vi "Msg Receive.vi"(11 "Self Actor in":refnum<class "Self Actor.lvclass">) -> (0 "error out":errorcluster, 2 "Destroy Self?":bool, 3 "Msg Receive out":refnum<class "Msg Receive.lvclass">)   [LabVIEW 2021, in "AAM.lvlib" / "Self Actor.lvclass"]
uses:
  Self Actor.lvclass
  C:/PPLs/LabVIEW-Composed-Actor-Model-LVCAM/LabVIEW-Composed-Actor-Model-LVCAM/AAM/AAM/Actor/Actor.lvclass
  Msg Receive/Msg Receive.lvclass
  Self Actor.lvclass/Self Actor.ctl
  Actor/Actor.lvclass
  C:/PPLs/LabVIEW-Composed-Actor-Model-LVCAM/LabVIEW-Composed-Actor-Model-LVCAM/AAM/AAM/Msg Receive/Msg Receive.lvclass
  Msg/Msg.lvclass
  Msg Q/Msg Q.lvclass
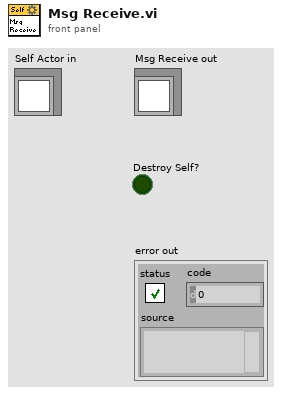
[diagram p1: front panel]
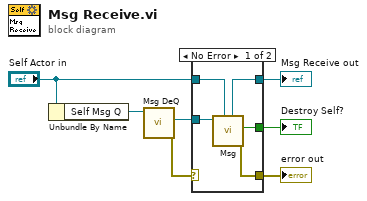
[diagram p0: block diagram]
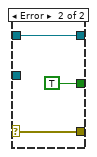
[diagram p2: hidden frame]
diagram:
  n1 = Unbundle By Name("Self Actor in") -> ("Self Msg Q"=w5:refnum<class "Msg Q.lvclass">)
  n2 = call "Msg DeQ.vi"("Msg Queue in"=w5) -> ("error out"=w6:errorcluster, "Msg"=w7:refnum<class "Msg.lvclass">)  [unwired: 9 in]
  n3 = case shown="No Error" w6 {
    selector: w6 -> [_ w14]
    tunnel: [w12 TRUE ("Destroy Self?")] -> w2
    tunnel: [w11 w14] -> w3
    tunnel: [w9 w15] -> w1
    tunnel: "Self Actor in" -> [w8 w15]
    tunnel: w7 -> [w10 _]
    frame No Error {
      n4 = call-dynamic "Msg.vi"("Actor in"=w8, "Msg in"=w10) -> ("error out"=w11:errorcluster, "Destroy Self?"=w12:bool, "Actor out"=w9:refnum<class "Actor.lvclass">)  [unwired: 7 in]
    }
    frame Error {
    }
  }
  "error out" <- w3
  "Destroy Self?" <- w2
  "Msg Receive out" <- w1
